vi "Stop_Action.vi"(8 "error in":errorcluster caption="错误输入（无错误）") -> (0 "error out":errorcluster caption="错误输出")   [LabVIEW 2013]
uses:
  GlobValue.vi
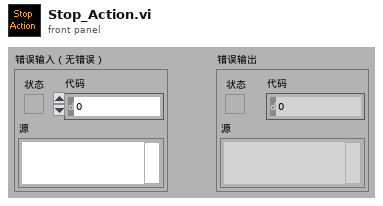
[diagram p1: front panel]
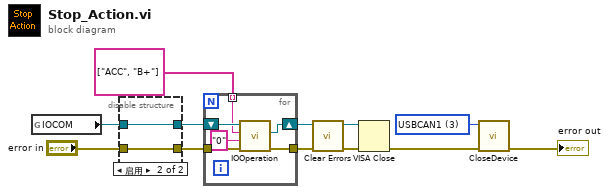
[diagram p0: block diagram]
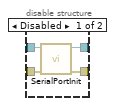
[diagram p2: hidden frame]
diagram:
  w10 = u32 3 items=["PCI5121"=1, "PCI9810"=2, "USBCAN1"=3, "USBCAN2"=4, "PCI9820"=5, "PCI5110"=7, "PC104CAN"=11, "CANETUDP"=12, "PCI9840B"=14, "PC104C2"=15, "PCI9820I"=16, "CANETTCP"=17, "PCIE9221"=24, "PCI5010U"=19, "USBCAN_E_U"=20, "USBCAN_2E_U"=21, "PCI5020U"=22] ("设备类型")
  n1 = global read "GlobValue.vi" "IOCOM"() -> (w8:refnum<visa-resource-name>)
  n2 = disable-structure shown="启用" {
    disable-tunnel: w8 -> [w15 w17]
    disable-tunnel: [w14 w17] -> w7
    disable-tunnel: "error in" -> [w13 w16]
    disable-tunnel: [w12 w16] -> w5
    frame Disabled {
      n3 = call "SerialPortInit.vi"("错误输入"=w13, "COMIn"=w15) -> ("错误输出"=w12:errorcluster, "COMOut"=w14:refnum<visa-resource-name>)  [unwired: 8 in]
    }
    frame Enabled {
    }
  }
  n4 = for {
    tunnel: [w23] -> w9
    tunnel: w5 -> [w21]
    tunnel: string[] ["ACC", "B+"] -> [w20] mode=indexing
    shift-right: [w18] -> w2
    shift-left: w7 -> [w22]
    n5 = call "IOOperation.vi"("error in"=w21, "Value"="0", "Channel"=w20, "Com"=w22) -> ("error out"=w23:errorcluster, "ComOut"=w18:refnum<visa-resource-name>)  [unwired: 5 in, 1 out]
  }
  n6 = call <vilib>:"Clear Errors.vi"("error in (no error)"=w9) -> ("error out"=w1:errorcluster)  [unwired: 6 in]
  n7 = VISA Close(VISA resource name=w2, error in (no error)=w1) -> (error out=w3:errorcluster)
  n8 = call "CloseDevice.vi"("错误输入（无错误）"=w3, "设备类型"=w10) -> ("错误输出"=→"error out":errorcluster)  [unwired: 8 in, 1 out]
